vi "ConfigureAppender.vi"(7 "id":string, 8 "error in (no error)":errorcluster, 9 "filter":T1={"mode"=enum."Mirror", "levelMin"=enum."INFO", "levelMax"=enum."INFO", "tagPrefix"=""}, 10 "threshold":T3=enum."INFO", 11 "Logger in":refnum<class "Logger.lvclass">) -> (0 "error out":errorcluster, 3 "Logger out":refnum<class "Logger.lvclass">)   [LabVIEW 2026, in "Lumberjack.lvlib" / "Logger.lvclass"]
uses:
  Logger.lvclass
  TypeDefs/Severity.ctl
  TypeDefs/Filter.ctl
  TypeDefs/FilterMode.ctl
  Logger.lvclass/Logger.ctl
  <vilib>/ActorFramework/Message Enqueuer/Message Enqueuer.lvclass
  Core/Messages/ConfigureAppenderMsg.lvclass/ConfigureAppenderMsg.lvclass
  Lumberjack.lvlib
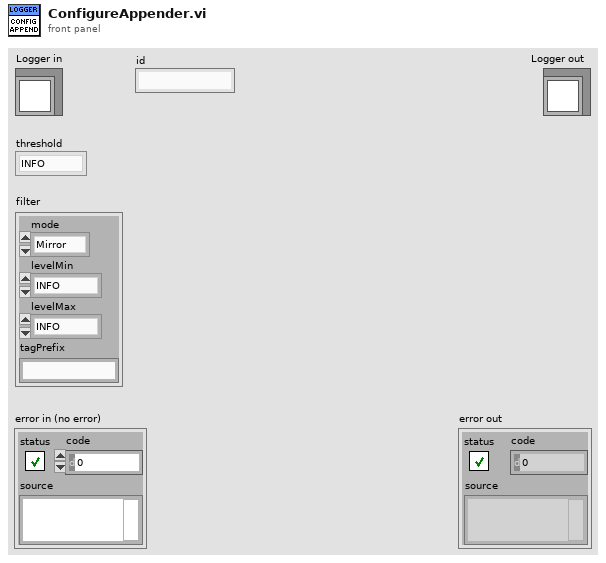
[diagram p1: front panel]
types:
  T1 = typedef "Lumberjack.lvlib/Filter.ctl" = cluster{"mode":T2, "levelMin":T3, "levelMax":T3, "tagPrefix":string}
  T2 = typedef "Lumberjack.lvlib/FilterMode.ctl" = enum16{"Mirror", "Routed"}
  T3 = typedef "Lumberjack.lvlib/Severity.ctl" = enum16{"OFF", "FATAL", "ERROR", "WARN", "INFO", "DEBUG", "TRACE", "ALL"}
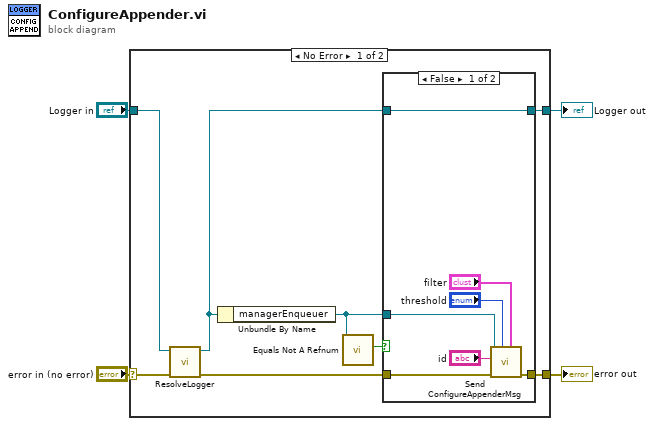
[diagram p0: block diagram]
diagram:
  n1 = case shown="No Error" "error in (no error)" {
    selector: "error in (no error)" -> [w12 w23]
    tunnel: [w10 w23] -> w3
    tunnel: [w8 w22] -> w1
    tunnel: "Logger in" -> [w9 w22]
    frame No Error {
      n2 = call "ResolveLogger.vi"("error in (no error)"=w12, "Logger in"=w9) -> ("error out"=w11:errorcluster, "Logger out"=w7:refnum<class "Logger.lvclass">)  [unwired: 8 in]
      n3 = Unbundle By Name(w7) -> ("managerEnqueuer"=w5:refnum<class "Message Enqueuer.lvclass">)
      n4 = call <vilib>:"Equals Not A Refnum.vi"("Message Enqueuer"=w5) -> ("Not a refnum?"=w6:bool)  [unwired: 10 in]
      n5 = case shown="False" w6 {
        tunnel: w11 -> [w19 w21]
        tunnel: [w18 w21] -> w10
        tunnel: [w17 w20] -> w8
        tunnel: w7 -> [w17 w20]
        tunnel: w5 -> [w16 _]
        frame False {
          n6 = call "Send ConfigureAppenderMsg.vi"("filter"="filter", "threshold"="threshold", "error in (no error)"=w19, "id"="id", "Enqueuer in"=w16) -> ("error out"=w18:errorcluster)  [unwired: 5 in, 1 out]
        }
        frame True {
        }
      }
    }
    frame Error {
    }
  }
  "error out" <- w3
  "Logger out" <- w1
